vi "Emballage_BDD_LireNoArticleJDE.vi"(8 "error in":errorcluster, 11 "NO_CDEVAL":string) -> (0 "error out":errorcluster, 2 "Erreur de\n comunication":bool, 3 "NO_ARTICLE_JDE":string)   [LabVIEW 2020]
doc: "Liste les commandes relatives au produit à emballer dans la GPAO.\nRenvoie un tableau contenant :\n 0 - le n° article FAS (ex. 12-216C-04520)\n 1 - le n° FILE FAS (ex. F120023)\n 2 - la designation du produit (ex. 211mA 57ohm)\n 3 - le n° cmde FAS\n 4 - la quantité à emballer\n 5 - ID cmde\n 6 - le n° cmde client\n 7 - le nom du client\n 8 - n° article client\n 9 - indice revision client\n 10 - société de facturation\n 11 - langue à utiliser\n 12 - retour? 0 non, 1 oui"
uses:
  Modules/FS/60_FS_Controles/60_FS_SetGet.ctl
  <vilib>/addons/database/Connection.llb/DB Tools Open Connec (Path).vi
  <vilib>/addons/database/NI_Database_API.lvlib
panel:
  out "temps Exe [s]":dbl
  out "requete":string="where (NO_ARTICLE ='12-216C-04521') and (NO_FILE ='EQIFIL') and (DESIGNATION LIKE '%104mA%')"
  in  "Table com":string="V_P_LIGCDEVAL"
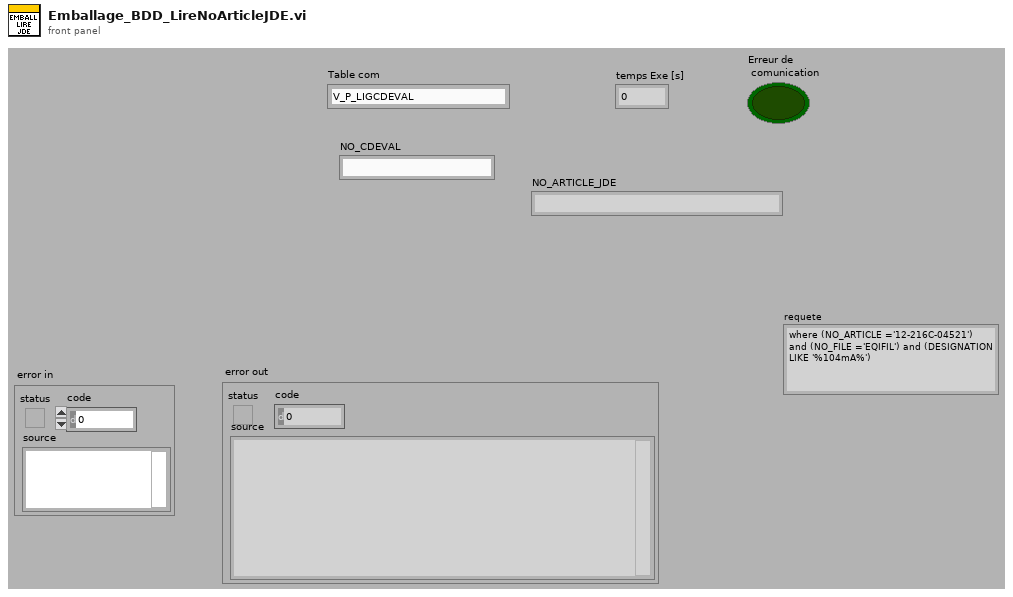
[diagram p1: front panel]
types:
  T1 = typedef "60_FS_SetGet.ctl" = enum16{"set", "get"}
  T2 = typedef "60_FS_CLT_Chemins.ctl" = cluster{"Racine_local":path, "Racine_reseau":path, "Racine_Support_Application":path, "Fichier_Journalisation":path, "Connexion_BDD_VSX":path, "Connexion_BDD_PLZ":path}
  T3 = typedef "NI_Database_API.lvlib/Conn ObjectReference.ctl" = refnum<k1>
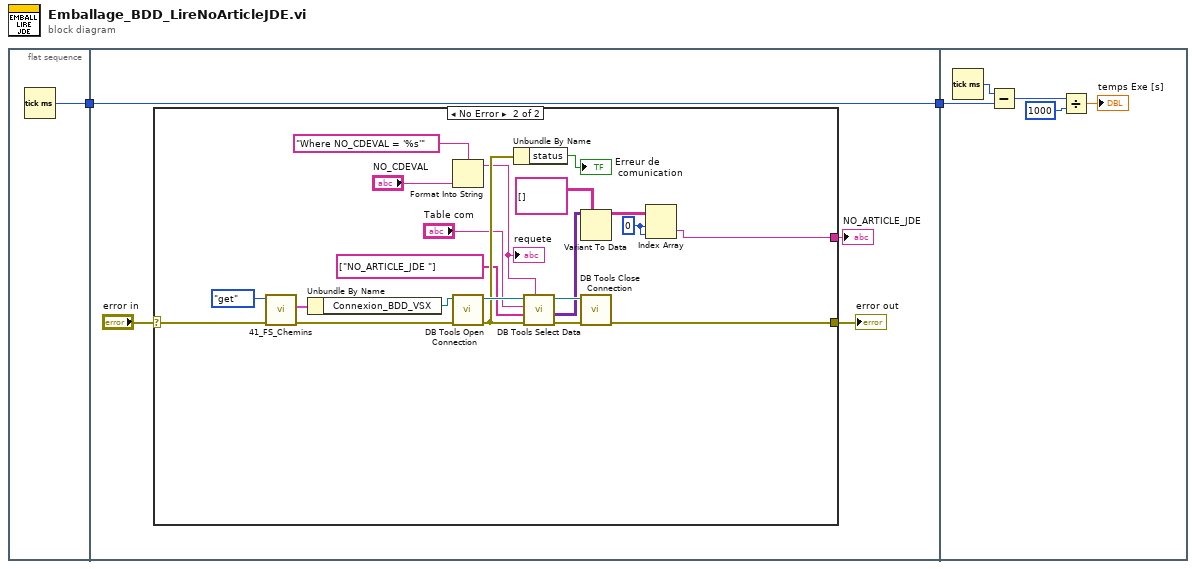
[diagram p0: block diagram]
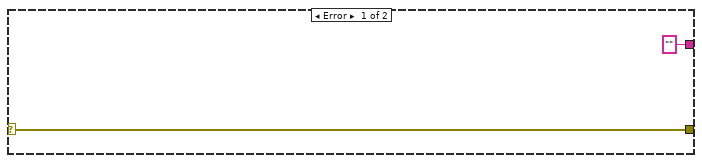
[diagram p2: hidden frame]
diagram:
  n1 = flat-sequence {
    tunnel: [w3] -> w1
    tunnel: [w5] -> w2
    tunnel: w1 -> [w5]
    tunnel: w2 -> [w31]
    frame #0 {
      n2 = Tick Count (ms)() -> (millisecond timer value=w3:u32)
    }
    frame #1 {
      n3 = case shown="No Error" "error in" {
        selector: "error in" -> [w9 w27]
        tunnel: [w9 w24] -> w7
        tunnel: ["" ("String") w10] -> w4
        frame Error {
        }
        frame No Error {
          w11 = 0 ("indice (ligne)")
          n4 = call "41_FS_Chemins.vi"("error in (no error)"=w27, "SetGet"=60_FS_SetGet."get") -> ("error out"=w26:errorcluster, "CLT_Chemins_out"=w29:T2)  [unwired: 8 in]
          n5 = Unbundle By Name(w29) -> ("Connexion_BDD_VSX"=w25:path)
          n6 = Format Into String(format string="Where NO_CDEVAL = '%s'" ("condition"), "NO_CDEVAL") -> (resulting string=w15:string)  [unwired: 2 in, 1 out]
          "requete" <- w15
          n7 = call-poly <vilib>:"DB Tools Open Connection.vi"("error in (no error)"=w26, "connection information"=w25) -> ("error out"=w22:errorcluster, "connection reference"=w23:T3)  [unwired: 6 in]
          n8 = Unbundle By Name(w22) -> ("status"=→"Erreur de\n comunication":bool)
          n9 = call <vilib>:"DB Tools Select Data.vi"("condition"=w15, "error in (no error)"=w22, "columns"=string[] ["NO_ARTICLE_JDE "], "table"="Table com", "connection reference"=w23) -> ("error out"=w20:errorcluster, "data"=w13:variant[][], "connection reference out"=w19:T3)  [unwired: 1 in]
          n10 = Variant To Data(type=string[][] [] ("Liste des champs à lire 2"), Variant=w13) -> (data=w12:string[][])  [unwired: 1 in, 1 out]
          n11 = call <vilib>:"DB Tools Close Connection.vi"("error in (no error)"=w20, "connection reference"=w19) -> ("error out"=w24:errorcluster)  [unwired: 5 in]
          n12 = Index Array(array=w12, index (row)=w11, index (col)=w11) -> (element=w10:string)
        }
      }
      "error out" <- w7
      "NO_ARTICLE_JDE" <- w4
    }
    frame #2 {
      n13 = Tick Count (ms)() -> (millisecond timer value=w35:u32)
      n14 = Subtract(x=w35, y=w31) -> (x-y=w32:u32)
      n15 = Divide(x=w32, y=u32 1000) -> (x/y=→"temps Exe [s]":dbl)
    }
  }
